vi "survo.vi"() -> ()   [LabVIEW 2016]
uses:
  <vilib>/DAQmx/write.llb/DAQmx Write (Digital 1D Bool NChan 1Samp 1Line).vi
  <vilib>/DAQmx/miscellaneous.llb/DAQmx Fill In Error Info.vi
panel:
  out "Data 3":bool[](array[boolean])
  out "Data 2":bool[](array[boolean])
  in  "stop":bool
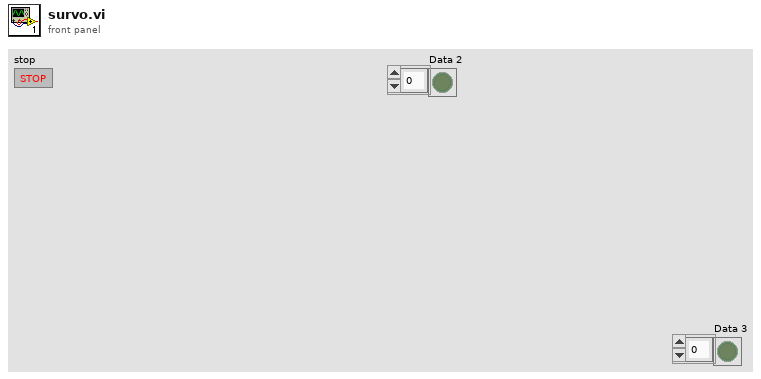
[diagram p1: front panel]
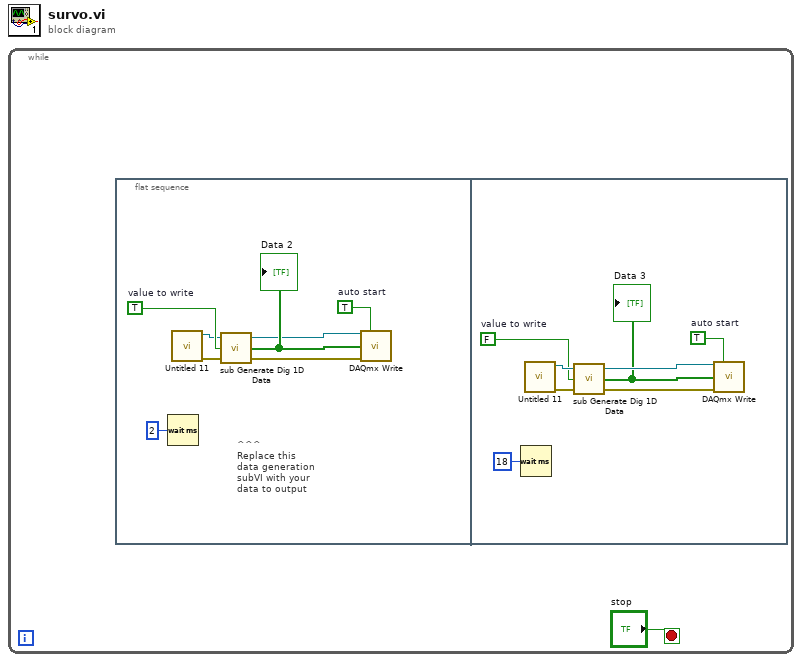
[diagram p0: block diagram]
diagram:
  n1 = while {
    stop <- "stop" stop-if-true
    n2 = flat-sequence {
      frame #0 {
        w8 = TRUE  # value to write
        w9 = TRUE  # auto start
        # "^^^\nReplace this\ndata generation\nsubVI with your\ndata to output"
        n3 = Wait (ms)(milliseconds to wait=u32 2) -> ()  [unwired: 1 out]
        n4 = call "Untitled 11.vi"() -> ("error out"=w3:errorcluster, "task out"=w4:refnum<k21>)  [unwired: 10 in]
        n5 = call <vilib>:"sub Generate Dig 1D Data.vi"("error in"=w3, "initial value"=w8, "task in"=w4) -> ("error out"=w7:errorcluster, "Data"=w6:bool[], "task out"=w5:refnum<k21>)
        "Data 2" <- w6
        n6 = call-poly <vilib>:"DAQmx Write.vi"("task/channels in"=w5, "auto start"=w9, "data"=w6, "error in"=w7) -> ()  [unwired: 9 in, 3 out]
      }
      frame #1 {
        w11 = FALSE  # value to write
        w10 = TRUE  # auto start
        n7 = Wait (ms)(milliseconds to wait=u32 18) -> ()  [unwired: 1 out]
        n8 = call "Untitled 11.vi"() -> ("error out"=w16:errorcluster, "task out"=w15:refnum<k21>)  [unwired: 10 in]
        n9 = call <vilib>:"sub Generate Dig 1D Data.vi"("error in"=w16, "initial value"=w11, "task in"=w15) -> ("error out"=w12:errorcluster, "Data"=w13:bool[], "task out"=w14:refnum<k21>)
        "Data 3" <- w13
        n10 = call-poly <vilib>:"DAQmx Write.vi"("task/channels in"=w14, "auto start"=w10, "data"=w13, "error in"=w12) -> ()  [unwired: 9 in, 3 out]
      }
    }
  }
